vi "LIN EX Master Read.vi"(7 "pData":u8[](array[numeric])=[0, 0, 0, 0, 0, 0, 0, 0], 8 "error in (no error)":errorcluster, 9 "PID":u8, 10 "LINIndex":u8, 11 "DevHandle":i32) -> (0 "error out":errorcluster, 3 "function return":i32, 5 "pData out":u8[](array[numeric]))   [LabVIEW 2010, in "usb2lin_ex.lvlib"]
doc: "int WINAPI LIN_EX_MasterRead(int DevHandle,unsigned char LINIndex,unsigned char PID,unsigned char *pData);"
uses:
  usb2lin_ex.lvlib
  USB2XXX/trunk/USB2XXX/USB2XXX/vs2010/Release/USB2XXX.dll
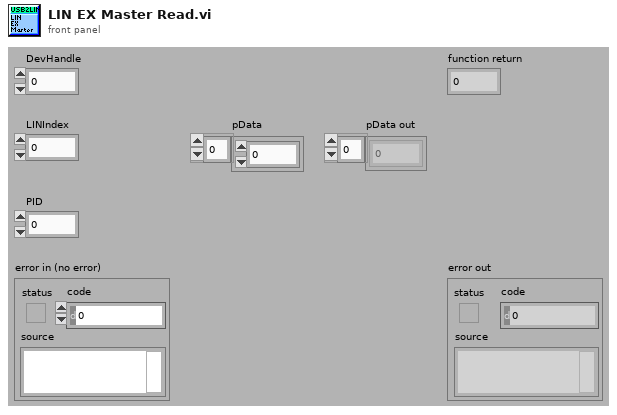
[diagram p1: front panel]
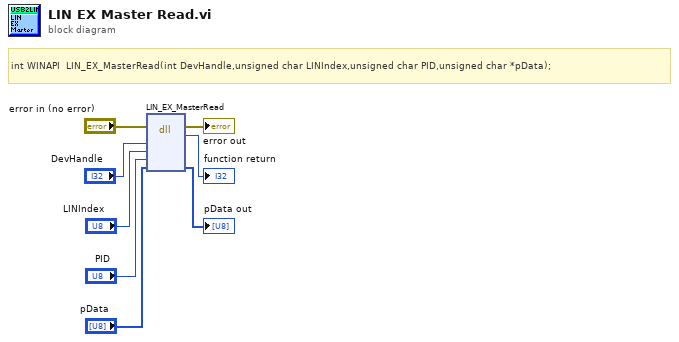
[diagram p0: block diagram]
diagram:
  # "int WINAPI  LIN_EX_MasterRead(int DevHandle,unsigned char LINIndex,unsigned char PID,unsigned char *pData);"
  n1 = dll-call lib="E:/OtherWork/STM32/USB2XXX/trunk/USB2XXX/USB2XXX/vs2010/Release/USB2XXX.*" fn="LIN_EX_MasterRead"(error in="error in (no error)", "DevHandle"="DevHandle", "LINIndex"="LINIndex", "PID"="PID", "pData"="pData") -> (error out=→"error out":errorcluster, →"function return":i32, "pData"=→"pData out":u8[])  [unwired: 5 in, 1 out]
